vi "worksheet activate.vi"(8 "error in (no error)":errorcluster, 11 "worksheet":u32) -> (0 "error out":errorcluster)   [LabVIEW 2015, in "xlsxwriter.lvlib"]
doc: "void worksheet_activate(lxw_worksheet worksheet);"
uses:
  xlsxwriter.lvlib
  xlsxwriter.dll
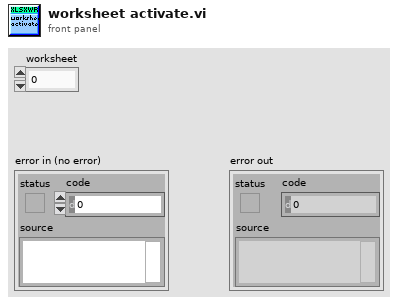
[diagram p1: front panel]
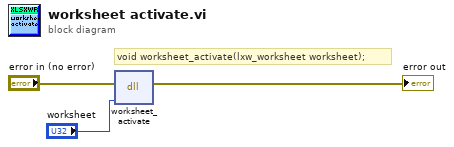
[diagram p0: block diagram]
diagram:
  # "void worksheet_activate(lxw_worksheet worksheet);"
  n1 = dll-call lib="C:/Users/WDAGUtilityAccount/Desktop/lv_vis_added_cell/xlsxwriter.*" fn="worksheet_activate"(error in="error in (no error)", "worksheet"="worksheet") -> (error out=→"error out":errorcluster)  [unwired: 4 in, 1 out]
